vi "Main_10A.vi"() -> ()   [LabVIEW 2024]
uses:
  Utility/Universal Utility/TypeDefs_Utility/Cluster_Row-Column.ctl
  Utility/Universal Utility/TypeDefs_Utility/ENUM_4 Directions U-D-L-R.ctl
panel:
  out "Paths":i32[](array[numeric])
  out "Array 2":i32[][](array[numeric])
  in  "Use Puzzle":bool
  out "Answer 652":u32
  in  "Puzzle":string="7651234510103430129656654566543012101234544567676545\n8340987643212345038743783087452143450925655438585432\n9205676544569416545032192196567854567810710129891201\n0114323456678507896123010105432945498789878778100323\n1023210987897612387654981234941834354308909689011414\n4321301010767887434767876547870921267210218574326505\n5650452121456996545897987676589810898876123465467876\n4781965432348765698018734585476701017965019894894966\n9890874321089450367129653090365432676874320767743987\n0781103016567321458934532101270121085401221678652156\n1692012923498212367012983501989789098320034569565043\n25431278743210034..."
  in  "Example":string="89010123\n78121874\n87430965\n96549874\n45678903\n32019012\n01329801\n10456732"
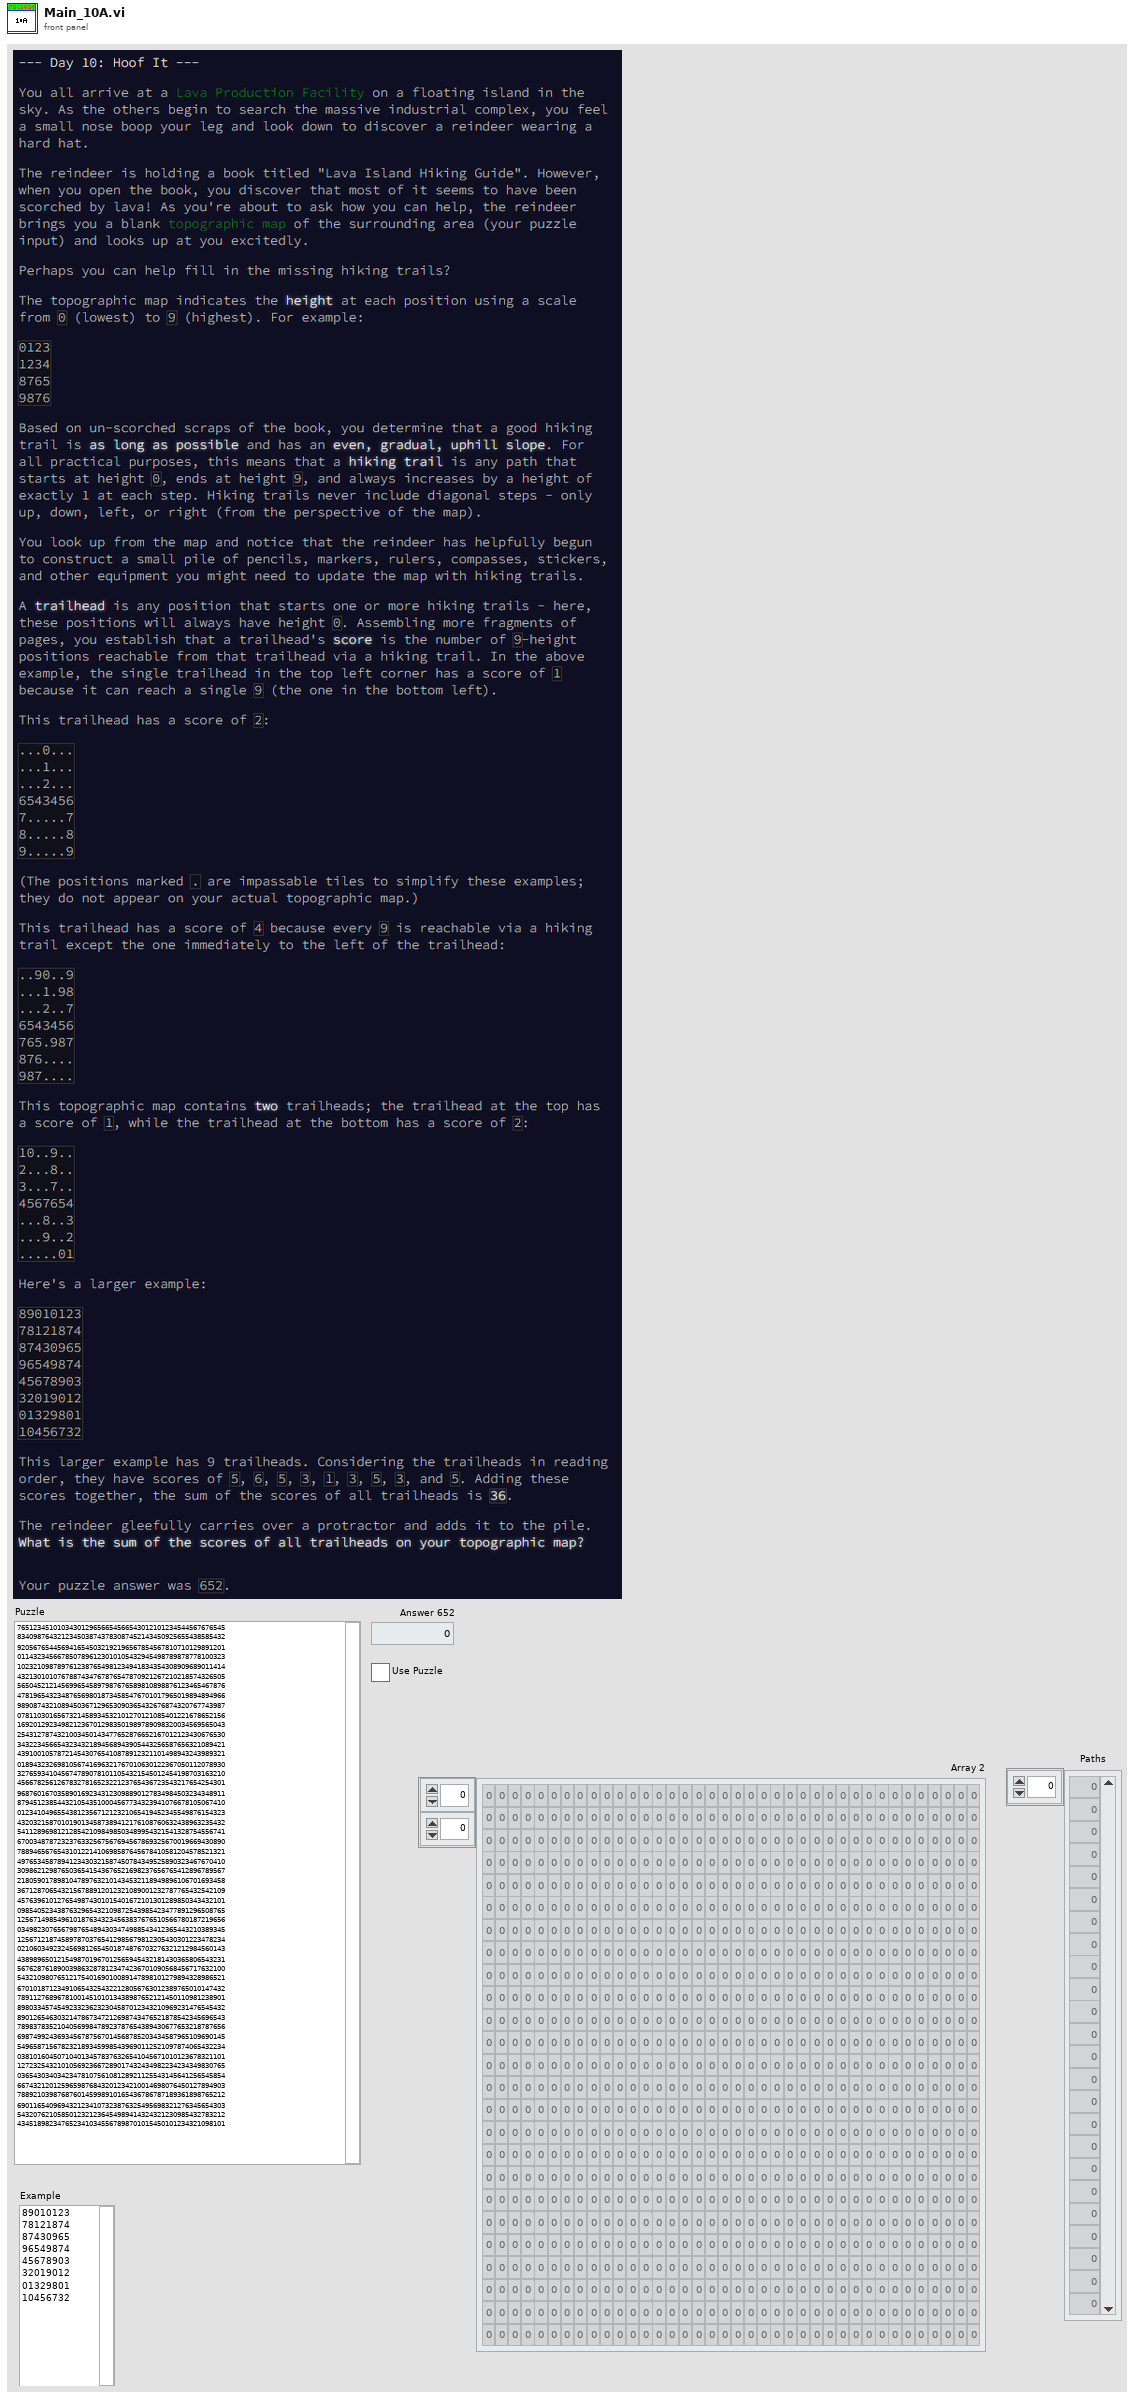
[diagram p1: front panel]
types:
  T1 = typedef "Cluster_Row-Column.ctl" = cluster{"R":i32, "C":i32}
  T2 = typedef "ENUM_4 Directions U-D-L-R.ctl" = enum16{"Up;-1,0", "Right;0,1", "Down;1,0", "Left;0,-1"}
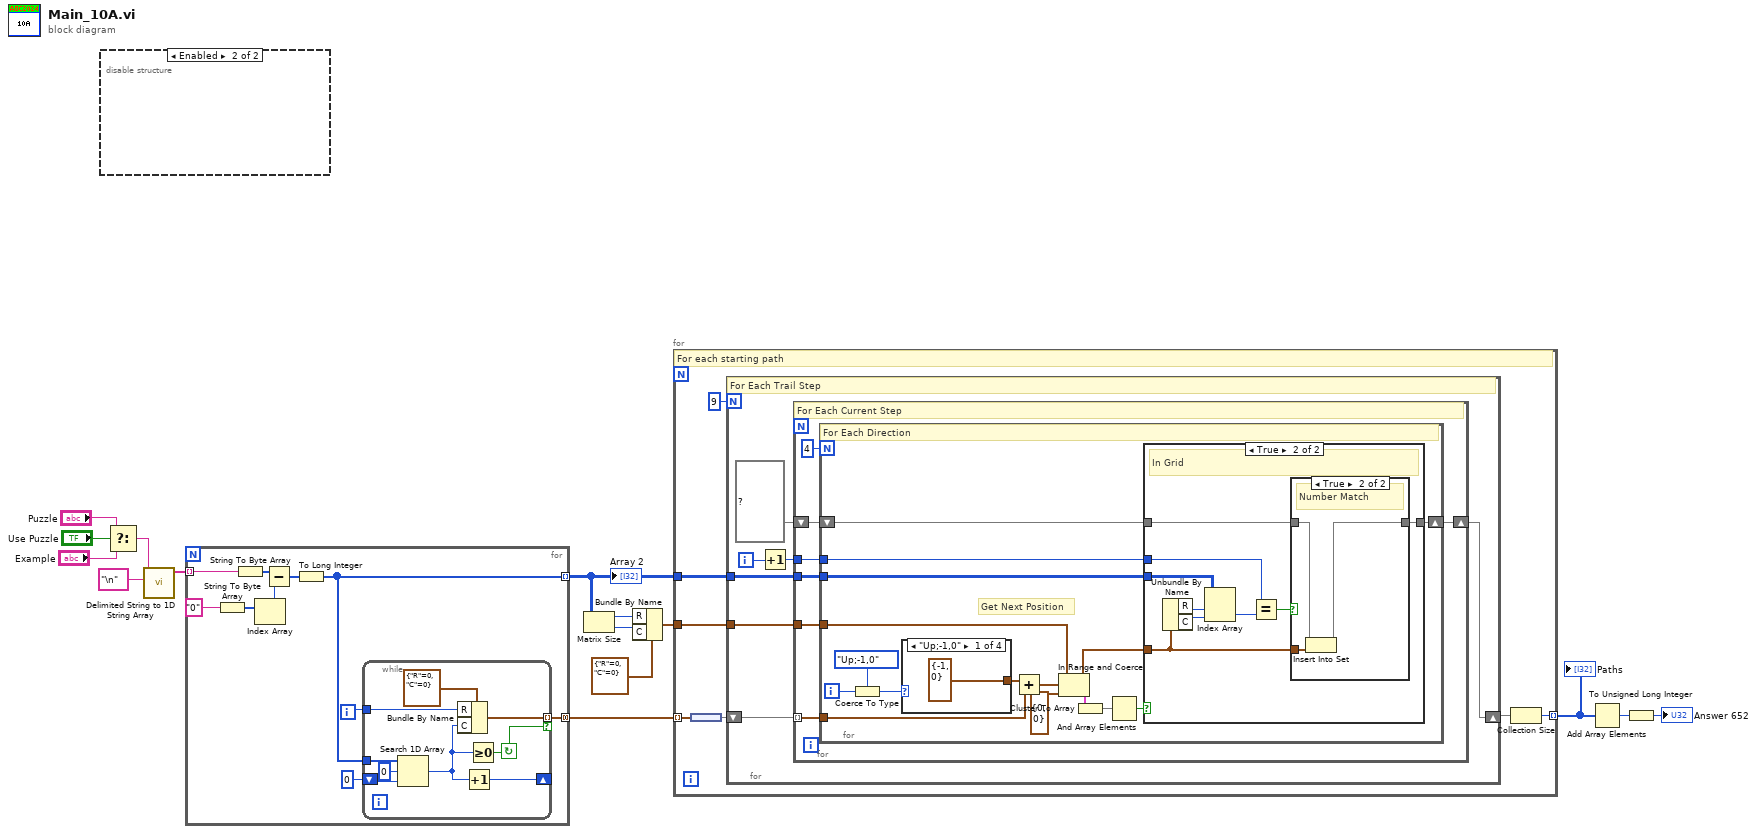
[diagram p0: block diagram]
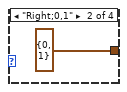
[diagram p4: hidden frame]
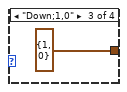
[diagram p5: hidden frame]
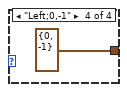
[diagram p6: hidden frame]
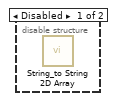
[diagram p7: hidden frame]
diagram:
  n1 = disable-structure shown="Enabled" {
    frame Disabled {
      n2 = call "String_to String 2D Array.vi"() -> ()  [unwired: 11 in, 1 out]
    }
    frame Enabled {
    }
  }
  n3 = Select(t="Puzzle", s="Use Puzzle", f="Example") -> (s? t:f=w13:string)
  n4 = call <vilib>:"Delimited String to 1D String Array.vi"("delimiter"="\n" ("delimiter (Tab)"), "delimited string"=w13) -> ("string array"=w10:string[])  [unwired: 9 in]
  n5 = for {
    tunnel: w10 -> [w22] mode=indexing
    tunnel: [w16] -> w8 mode=indexing
    tunnel: [w19] -> w9 mode=concatenating
    i -> [w20]
    n6 = String To Byte Array(string="0") -> (unsigned byte array=w24:u8[])
    n7 = String To Byte Array(string=w22) -> (unsigned byte array=w21:u8[])
    n8 = Index Array(array=w24) -> (element=w23:u8)  [unwired: 1 in]
    n9 = Subtract(x=w21, y=w23) -> (x-y=w17:u8[])
    n10 = To Long Integer(number=w17) -> (32bit integer=w16:i32[])
    n11 = while {
      tunnel: w16 -> [w34]
      shift-right: [w32] -> _
      shift-left: 0 -> [w33]
      tunnel: w20 -> [w31]
      tunnel: [w29] -> w19 mode=indexing if=w28
      stop <- w28 continue-if-true
      n12 = Search 1D Array(1D array=w34, element=0, start index (0)=w33) -> (index of element=w30:i32)
      n13 = Bundle By Name(cluster=T1 {"R"=0, "C"=0} ("Position"), "R"=w31, "C"=w30) -> (w29:T1)
      n14 = Increment(x=w30) -> (x+1=w32:i32)
      n15 = Greater Or Equal To 0?(x=w30) -> (x >= 0?=w28:bool)
    }
  }
  "Array 2" <- w8
  n16 = Matrix Size(0:w8) -> (1:w6:i32, 2:w5:i32)
  n17 = Bundle By Name(cluster=T1 {"R"=0, "C"=0} ("Position"), "R"=w6, "C"=w5) -> (w4:T1)
  n18 = for {
    tunnel: w9 -> [w38] mode=indexing
    tunnel: w8 -> [w40]
    tunnel: w4 -> [w41]
    tunnel: [w35] -> w3 mode=indexing
    # "For each starting path"
    n19 = node(w38) -> (w37:set{T1})
    n20 = for {
      N: 9 -> [_]
      tunnel: w41 -> [w47]
      tunnel: w40 -> [w46]
      shift-right: [w44] -> w36
      shift-left: w37 -> [w48]
      i -> [w43]
      # "For Each Trail Step"
      n21 = Increment(x=w43) -> (x+1=w42:i32)
      n22 = for {
        tunnel: w48 -> [w55] mode=indexing
        tunnel: w47 -> [w54]
        tunnel: w46 -> [w53]
        shift-right: [w50] -> w44
        shift-left: set{T1} {} ("set") -> [w51]
        tunnel: w42 -> [w49]
        # "For Each Current Step"
        n23 = for {
          N: 4 -> [_]
          tunnel: w55 -> [w67]
          tunnel: w54 -> [w65]
          tunnel: w53 -> [w60]
          shift-right: [w57] -> w50
          shift-left: w51 -> [w58]
          tunnel: w49 -> [w56]
          i -> [w71]
          # "Get Next Position"
          # "For Each Direction"
          n24 = Coerce To Type(0:w71, 1:ENUM_4_Directions_U-D-L-R."Up;-1,0" ("Direction")) -> (2:w70:T2)
          n25 = case shown="\"Up;-1,0\"" w70 {
            tunnel: [T1 {"R"=-1, "C"=0} ("Position") T1 {"R"=0, "C"=1} ("Position") T1 {"R"=1, "C"=0} ("Position") T1 {"R"=0, "C"=-1} ("Position")] -> w68
            frame "Up;-1,0" {
            }
            frame "Right;0,1" {
            }
            frame "Down;1,0" {
            }
            frame "Left;0,-1" {
            }
          }
          n26 = Add(x=w68, y=w67) -> (x+y=w66:T1)
          n27 = In Range and Coerce(upper limit=w65, x=w66, lower limit=T1 {"R"=0, "C"=0}) -> (coerced(x)=w59:T1, In Range?=w63:cluster{"R":bool, "C":bool})
          n28 = Cluster To Array(cluster=w63) -> (array=w62:bool[])
          n29 = And Array Elements(Boolean array=w62) -> (logical AND=w61:bool)
          n30 = case shown="True" w61 {
            tunnel: w60 -> [_ w81]
            tunnel: w59 -> [_ w73]
            tunnel: w56 -> [_ w77]
            tunnel: w58 -> [w72 w75]
            tunnel: [w72 w74] -> w57
            frame False {
              # "Out of Grid"
            }
            frame True {
              # "In Grid"
              n31 = Unbundle By Name(w73) -> ("R"=w80:i32, "C"=w79:i32)
              n32 = Index Array(array=w81, index (row)=w80, index (col)=w79) -> (element=w78:i32)
              n33 = Equal?(x=w77, y=w78) -> (x = y?=w76:bool)
              n34 = case shown="True" w76 {
                tunnel: w75 -> [w82 w85]
                tunnel: [w82 w84] -> w74
                tunnel: w73 -> [_ w83]
                frame False {
                  # "No Match"
                }
                frame True {
                  # "Number Match"
                  n35 = Insert Into Set(10:w83, 11:w85) -> (3:w84:set{T1})  [unwired: 1 out]
                }
              }
            }
          }
        }
      }
    }
    n36 = Collection Size(1:w36) -> (0:w35:i32)
  }
  "Paths" <- w3
  n37 = Add Array Elements(numeric array=w3) -> (sum=w1:i32)
  n38 = To Unsigned Long Integer(number=w1) -> (unsigned 32bit integer=→"Answer 652":u32)
